vi "Demo Play wav file to Sound Output.vi"(10 "Number of Samples/Iteration":i32=50000, 11 "File Path":path) -> ()   [LabVIEW 2011]
doc: "This VI illustrates how to play a sound file continuously, reading the sound file in pieces, and playing each piece at a time."
uses:
  VIremote.llb/VIremoteFunction.ctl
  <vilib>/sound2/lvsound2.llb/Sound File Info (path).vi
  <vilib>/sound2/lvsound2.llb/Sound File Read Open.vi
  <vilib>/sound2/lvsound2.llb/Sound File Read (I16).vi
panel:
  out "error out":errorcluster
  in  "error in (no error)":errorcluster
  out "Loop Index":i32
  # "This VI plays a wav sound file continuously, reading the sound file in pieces, and playing each piece at a time."
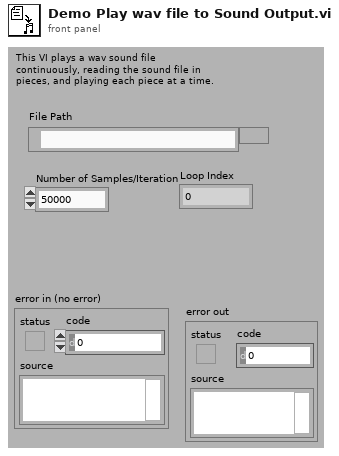
[diagram p1: front panel]
types:
  T1 = typedef "VIremoteFunction.ctl" = enum16{"Do nothing", "Stop controller", "Close this connection", "Show info panel", "Set VI to control", "Set Accelerometer freq (Hz)", "Show Alert message", "Start Sound Input", "Stop Sound Input", "Set Volume (0-100)", "Set sound output Speaker", "Set sound output Receiver", "Play Sound", "Repeat Sound", "Stop Sound", "Pause Sound", "Resume Sound", "Set panel width of caller (320 or 480)", "Set Panel Size to Portrait", "Set Panel Size to Landscape", "Set Panel Size as Current Orientation", "Allow all UI Orientations", "Send user notification", "Disable Scrolling", "Normal Scrolling", "Page Scrolling", "Set Scroll Offset", "Page Indicator Position"}
  T2 = cluster{"UIorientation":refnum<notifier>, "Accelerometer":refnum<notifier>, "Sound":refnum<notifier>, "SoundPlayBufferReady":refnum<notifier>, "BackgroundState":refnum<notifier>, "Touch":refnum<notifier>}
  T3 = typedef "Sound File Refnum.ctl" = refnum<file>
  T4 = enum16{"big-endian, network order", "native, host order", "little-endian"}
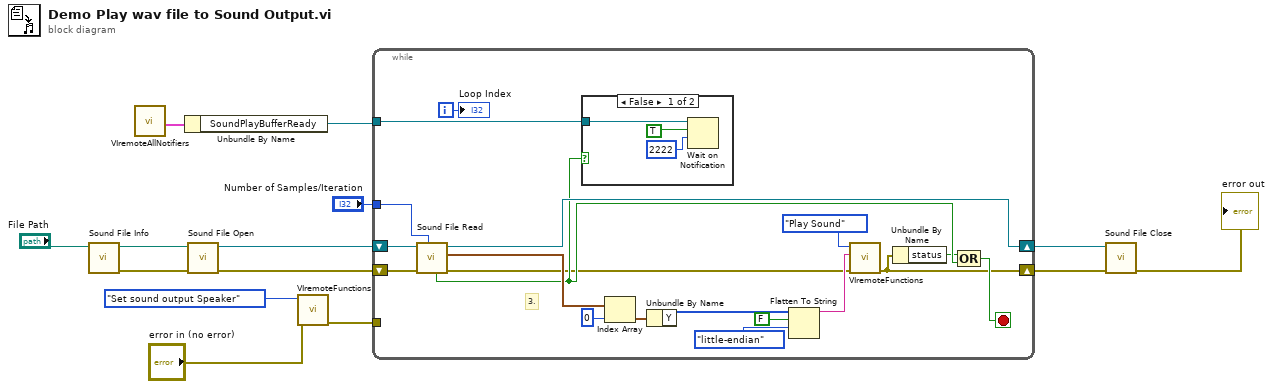
[diagram p0: block diagram]
diagram:
  n1 = call-poly <vilib>:"Sound File Info.vi"("path"="File Path") -> ("error out"=w11:errorcluster, "path out"=w10:path)  [unwired: 1 in, 8 out]
  n2 = call "VIremoteAllNotifiers.vi"() -> ("All Notifiers (unbundle by name)"=w8:T2)  [unwired: 1 in, 10 out]
  n3 = Unbundle By Name(w8) -> ("SoundPlayBufferReady"=w7:refnum<notifier>)
  n4 = call-poly <vilib>:"Sound File Open.vi"("error in (no error)"=w11, "path"=w10) -> ("error out"=w4:errorcluster, "sound file refnum"=w12:T3)  [unwired: 8 out]
  n5 = call "VIremoteFunctions.vi"("error in (no error)"="error in (no error)", "Function"=VIremoteFunction."Set sound output Speaker") -> ("error out"=w5:errorcluster)  [unwired: 4 in, 5 out]
  n6 = while {
    shift-right: [w21] -> w13
    shift-left: w4 -> [w33]
    tunnel: "Number of Samples/Iteration" -> [w28]
    shift-right: [w30] -> w14
    shift-left: w12 -> [w32]
    tunnel: w7 -> [w23]
    tunnel: w5 -> [_]
    i -> [w31]
    stop <- w29 stop-if-true
    # "3."
    n7 = call-poly <vilib>:"Sound File Read.vi"("number of samples/ch (-1: all)"=w28, "error in (no error)"=w33, "sound file refnum"=w32) -> ("error out"=w15:errorcluster, "data"=w26:waveform(i16)[], "sound file refnum out"=w30:T3, "end of file?"=w22:bool)  [unwired: 2 in, 3 out]
    n8 = case shown="False" w22 {
      tunnel: w23 -> [w36 _]
      frame False {
        n9 = Wait on Notification(notifier=w36, ignore previous (F)=TRUE, timeout in ms (-1)=2222) -> ()  [unwired: 1 in, 4 out]
      }
      frame True {
      }
    }
    n10 = Index Array(array=w26, index=0) -> (element=w25:waveform(i16))
    n11 = Unbundle By Name(w25) -> ("Y"=w17:i16[])
    n12 = Flatten To String(anything=w17, prepend array or string size? (T)=FALSE, byte order (0:big-endian, network order)=T4."little-endian") -> (data string=w16:string)  [unwired: 1 in, 2 out]
    n13 = call "VIremoteFunctions.vi"("error in (no error)"=w15, "String in"=w16, "Function"=VIremoteFunction."Play Sound") -> ("error out"=w21:errorcluster)  [unwired: 3 in, 5 out]
    n14 = Unbundle By Name(w21) -> ("status"=w20:bool)
    n15 = Compound Arithmetic op=OR(w20, w22) -> (w29:bool)
    "Loop Index" <- w31
  }
  n16 = call <vilib>:"Sound File Close.vi"("error in (no error)"=w13, "sound file refnum"=w14) -> ("error out"=→"error out":errorcluster)  [unwired: 9 out]
